vi "_AttributeInfo.vi"(0 "device name":string="unspecified value", 1 "min value":string="unspecified value", 2 "min alarm":string="unspecified value", 5 "attribute name":string="unspecified value", 7 "label":string="unspecified value", 9 "unit":string="unspecified value", 11 "display format":string="unspecified value", 12 "max value":string="unspecified value", 13 "max alarm":string="unspecified value") -> (8 "attribute info":T1)   [LabVIEW 2014, in "tango.lvlib"]
uses:
  tango.lvlib
  Common VIs/Typedefs/_AttributeInfo_t.ctl
  Common VIs/Typedefs/_AttributeAccess_t.ctl
  Common VIs/Typedefs/_AttributeFormat_t.ctl
  Common VIs/Typedefs/_TangoDataType_t.ctl
  Common VIs/Typedefs/_AttributeLevel_t.ctl
panel:
  # "AttributeInfo.r/w access\n-----------------------\n\tREAD = 0\n READ_WITH_WRITE = 1\n WRITE = 2\n READ_WRITE = 3"
  # "AttributeInfo.format\n-----------------------\n\tSCALAR = 0\n SPECTRUM = 1\n IMAGE = 2"
  # "AttributeInfo.level\n-----------------------\n\tOPERATOR = 0\n EXPERT = 1"
  # "AttributeInfo.data-type\n-----------------------\n\tDEV_VOID = 0\n\tDEV_BOOLEAN = 1\n\tDEV_SHORT = 2\n\tDEV_LONG = 3\n\tDEV_FLOAT = 4\n\tDEV_DOUBLE = 5\n\tDEV_USHORT = 6\n\tDEV_ULONG = 7\n\tDEV_STRING = 8\n\tDEVVAR_CHARARRAY = 9\n\tDEVVAR_SHORTARRAY = 10\n\tDEVVAR_LONGARRAY = 11\n\tDEVVAR_FLOATARRAY = 12\n\tDEVVAR_DOUBLEARRAY = 13\n\tDEVVAR_USHORTARRAY = 14\n\tDEVVAR_ULONGARRAY = 15\n\tDEVVAR_STRINGARRAY = 16\n\tDEVVAR_LONGSTRINGARRAY = 17\n\tDEVVAR_DOUBLESTRINGARRAY = 18\n\tDEV_STATE = 19\n\tCONST_DEV_STRING = 20\n\tDEVVAR_BOOLEANARRAY = 21\n\tDEV_UCHAR = 22\n\tDEV_LONG64 = 23\n\tDEV_ULONG64 = 24\n\tDEVVAR_LONG64ARRAY = 25\n\tDEVVAR_ULONG64ARRAY = 26\n\tDEV_INT = 27\n\tDEV_ENCODED = 28"
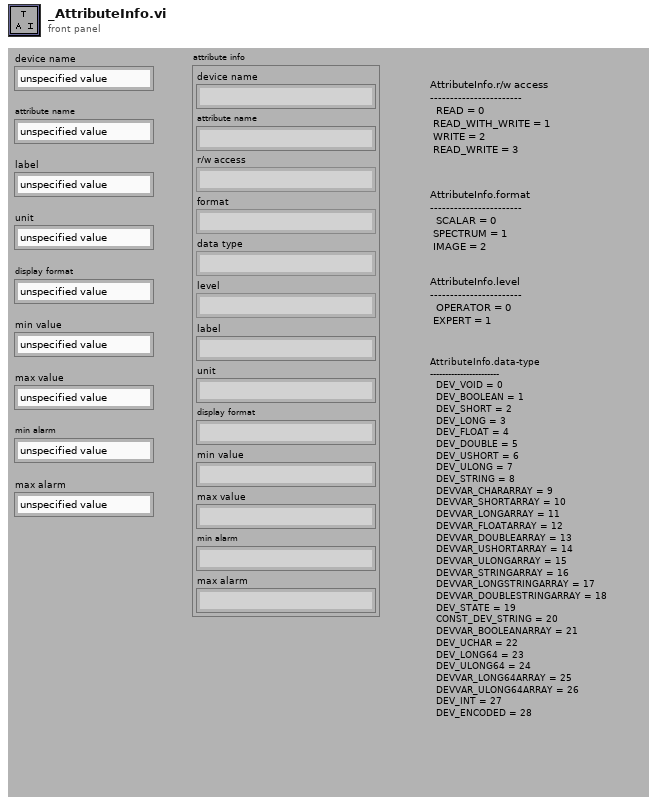
[diagram p1: front panel]
types:
  T1 = typedef "tango.lvlib/_AttributeInfo_t.ctl" = cluster{"device name":string, "attribute name":string, "r/w access":T2, "format":T3, "data type":T4, "level":T5, "label":string, "unit":string, "display format":string, "min value":string, "max value":string, "min alarm":string, "max alarm":string}
  T2 = typedef "tango.lvlib/_AttributeAccess_t.ctl" = enum16{"READ", "READ_WITH_WRITE", "WRITE", "READ_WRITE", "UNKNOWN_ACCESS_TYPE"}
  T3 = typedef "tango.lvlib/_AttributeFormat_t.ctl" = enum16{"SCALAR", "SPECTRUM", "IMAGE", "UNKNOWN_FORMAT"}
  T4 = typedef "tango.lvlib/_TangoDataType_t.ctl" = enum16{"VOID", "BOOLEAN", "SHORT", "LONG", "FLOAT", "DOUBLE", "USHORT", "ULONG", "STRING", "CHAR_ARRAY", "SHORT_ARRAY", "LONG_ARRAY", "FLOAT_ARRAY", "DOUBLE_ARRAY", "USHORT_ARRAY", "ULONG_ARRAY", "STRING_ARRAY", "LONG_STRING_ARRAY", "DOUBLE_STRING_ARRAY", "STATE", "CONST_STRING", "BOOLEAN_ARRAY", "UCHAR", "LONG64", "ULONG64", "LONG64_ARRAY", "ULONG64_ARRAY", "INT (not supported)", "ENCODED (not supported)", "ENUM", "PIPE_BLOB (not supported)", "STATE_ARRAY", "UNKNOW_DATA_TYPE"}
  T5 = typedef "tango.lvlib/_AttributeLevel_t.ctl" = enum16{"OPERATOR", "EXPERT", "UNKNOWN_LEVEL"}
  T6 = cluster{"device name":string, "attribute name":string, "r/w access":T2, "format":T3, "data type":T4, "level":T5, "label":string, "unit":string, "display format":string, "min value":string, "max value":string, "min alarm":string, "max alarm":string}
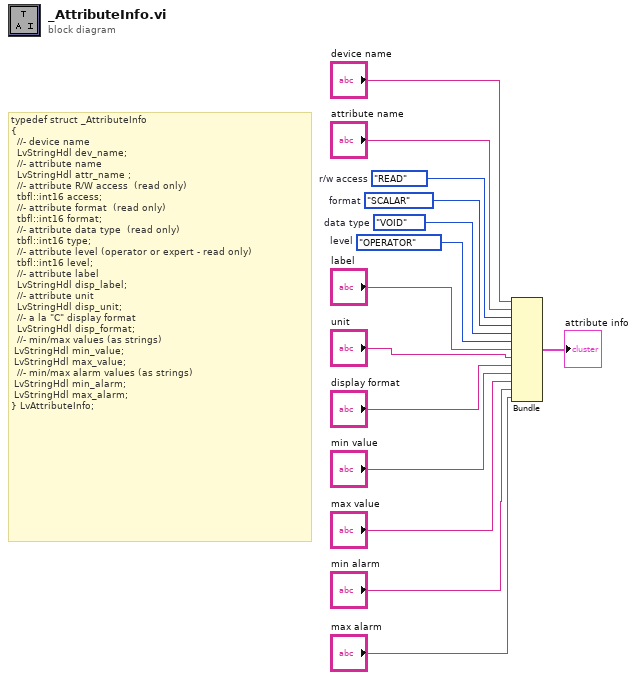
[diagram p0: block diagram]
diagram:
  w11 = _AttributeLevel_t."OPERATOR"  # level
  w12 = _TangoDataType_t."VOID"  # data type
  w13 = _AttributeFormat_t."SCALAR"  # format
  w14 = _AttributeAccess_t."READ"  # r/w access
  # "typedef struct _AttributeInfo\n{\n  //- device name\n  LvStringHdl dev_name;\n  //- attribute name \n  LvStringHdl attr_name ;\n  //- attribute R/W access  (read only)\n  tbfl::int16 access;\n  //- attribute format  (read only) \n  tbfl::int16 format;\n  //- attribute data type  (read only) \n  tbfl::int16 type;\n  //- attribute level (operator or expert - read only)\n  tbfl::int16 level;\n  //- attribute label\n  LvStringHdl disp_label;\n  //- attribute unit\n  LvStringHdl disp_unit;\n  //- a la \"C\" display format\n  LvStringHdl disp_format;\n  //- min/max values (as strings)\n\tLvStringHdl min_value;\n\tLvStringHdl max_value;\n  //- min/max alarm values (as strings)\n\tLvStringHdl min_alarm;\n\tLvStringHdl max_alarm;\n} LvAttributeInfo;"
  n1 = Bundle("device name"="device name", "attribute name"="attribute name", "r/w access"=w14, "format"=w13, "data type"=w12, "level"=w11, "label"="label", "unit"="unit", "display format"="display format", "min value"="min value", "max value"="max value", "min alarm"="min alarm", "max alarm"="max alarm") -> (→"attribute info":T6)  [unwired: 1 in]
